vi "room.vi"(7 "conti R3?":bool, 8 "error in (no error)":errorcluster, 9 "Position":T4, 10 "Enum":enum16{"recycle", "box put"}(ring), 11 "main.ctl":T1) -> (0 "error out":errorcluster, 1 "Position out":T4, 3 "main.ctl 2":T1)   [LabVIEW 2019]
uses:
  main data.ctl
  vision/vision_board_ctl.ctl
  block box.ctl
  subVI/move/position cluster.ctl
  servo state.ctl
  route_name.ctl
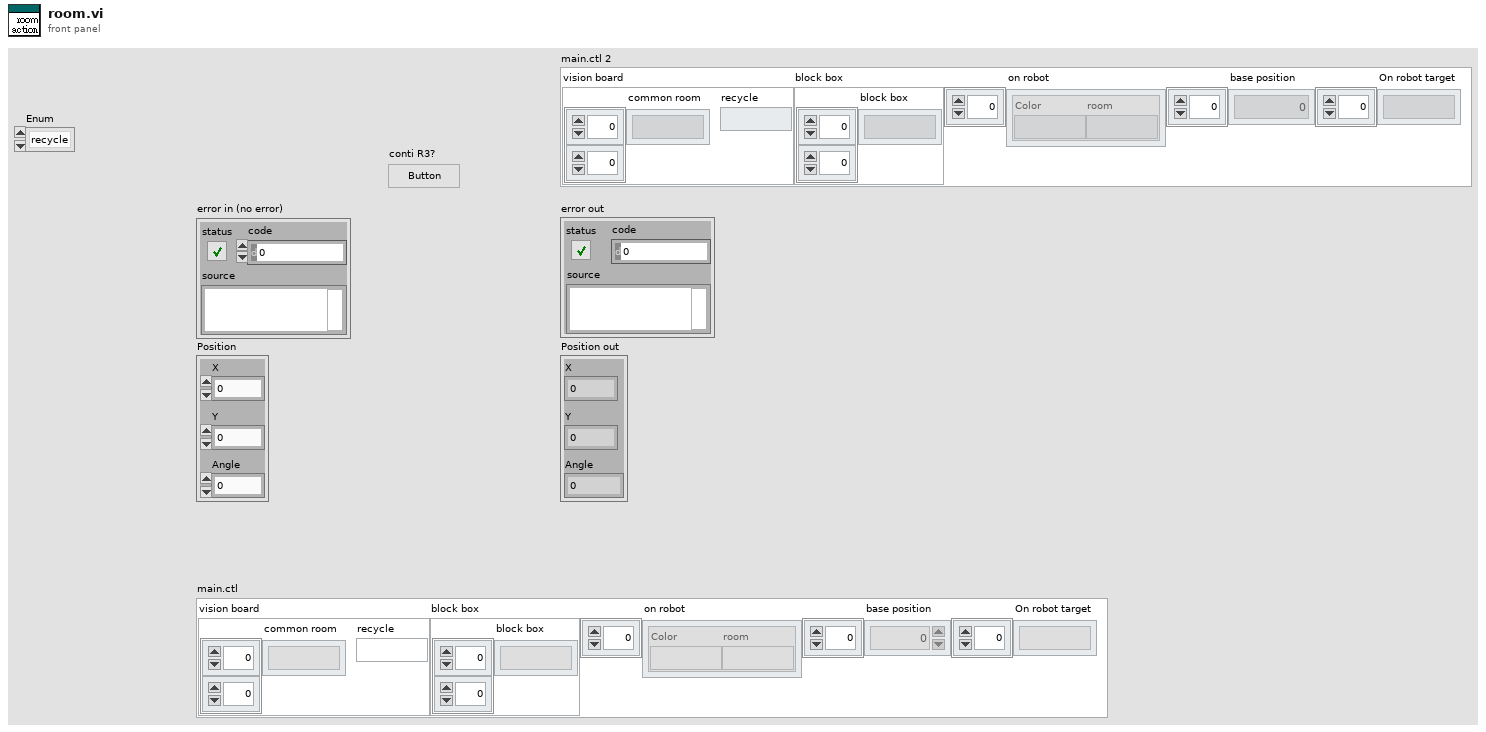
[diagram p1: front panel]
types:
  T1 = typedef "main data.ctl" = cluster{"vision board":T2, "block box":T3, "on robot ":cluster{"Color":string, "room":string}[], "base position":dbl[], "On robot target":string[]}
  T2 = typedef "vision_board_ctl.ctl" = cluster{"common room":string[][], "recycle":string}
  T3 = typedef "block box.ctl" = cluster{"block box":string[][]}
  T4 = typedef "position cluster.ctl" = cluster{"X":dbl, "Y":dbl, "Angle":dbl}
  T5 = typedef "route_name.ctl" = enum16{"S-Vision", "Vision-R1", "Vision-R2", "Vision-R3", "Vision-R4", "Vision-R5", "R1-Vision", "R2-Vision", "R3-Vision", "R4-Vision", "R5-Vision", "Vision-box", "box-recycle", "recycle-box", "box-Vision", "Vision-S", "R2-R3"}
  T6 = typedef "servo state.ctl" = enum16{"catch", "cam-1", "put", "side", "center", "side-2", "put-2"}
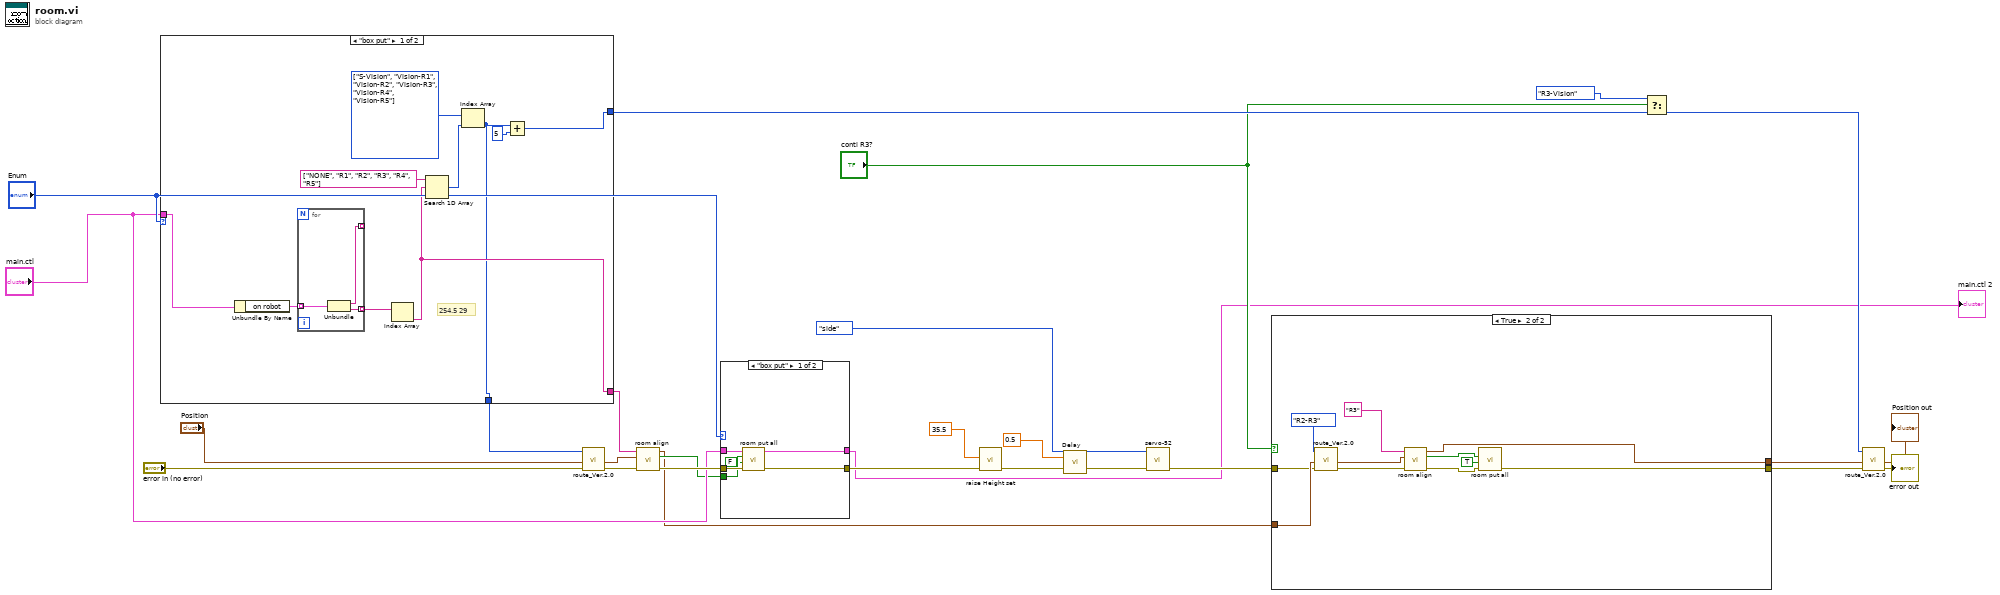
[diagram p0: block diagram]
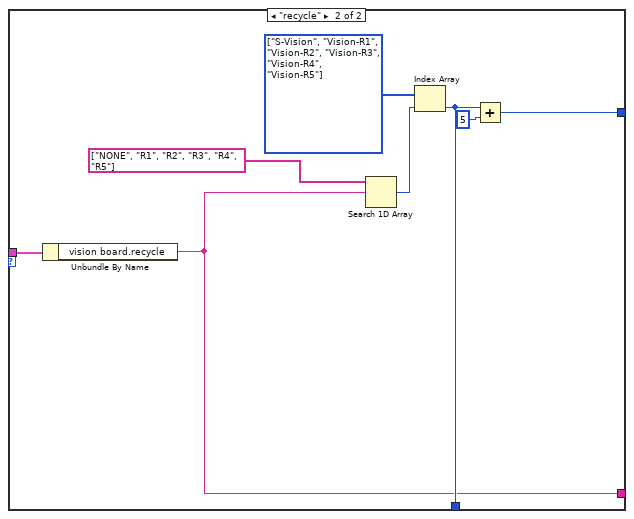
[diagram p3: hidden frame]
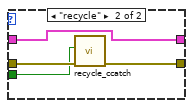
[diagram p4: hidden frame]
diagram:
  n1 = case shown="\"box put\"" "Enum" {
    tunnel: "main.ctl" -> [w28 w45]
    tunnel: [w29 w43] -> w27
    tunnel: [w30 w42] -> w24
    tunnel: [w31 w41] -> w21
    frame "box put" {
      w34 = T5[] [enum."S-Vision", enum."Vision-R1", enum."Vision-R2", enum."Vision-R3", enum."Vision-R4", enum."Vision-R5"] items=["S-Vision", "Vision-R1", "Vision-R2", "Vision-R3", "Vision-R4", "Vision-R5", "R1-Vision", "R2-Vision", "R3-Vision", "R4-Vision", "R5-Vision", "Vision-box", "box-recycle", "recycle-box", "box-Vision", "Vision-S", "R2-R3"]
      # "254.5 29"
      n2 = Unbundle By Name(w28) -> ("on robot"=w37:cluster{"Color":string, "room":string}[])
      n3 = for {
        tunnel: w37 -> [w40] mode=indexing
        tunnel: [w39] -> _ mode=indexing
        tunnel: [w38] -> w36 mode=indexing
        n4 = Unbundle(w40) -> ("Color"=w39:string, "room"=w38:string)
      }
      n5 = Index Array(array=w36) -> (element=w30:string)  [unwired: 1 in]
      n6 = Search 1D Array(1D array=string[] ["NONE", "R1", "R2", "R3", "R4", "R5"], element=w30) -> (index of element=w33:i32)  [unwired: 1 in]
      n7 = Index Array(array=w34, index=w33) -> (element=w29:T5)
      n8 = Add(x=w29, y=5) -> (x+y=w31:i32)
    }
    frame "recycle" {
      w47 = T5[] [enum."S-Vision", enum."Vision-R1", enum."Vision-R2", enum."Vision-R3", enum."Vision-R4", enum."Vision-R5"] items=["S-Vision", "Vision-R1", "Vision-R2", "Vision-R3", "Vision-R4", "Vision-R5", "R1-Vision", "R2-Vision", "R3-Vision", "R4-Vision", "R5-Vision", "Vision-box", "box-recycle", "recycle-box", "box-Vision", "Vision-S", "R2-R3"]
      n9 = Unbundle By Name(w45) -> ("vision board.recycle"=w42:string)
      n10 = Search 1D Array(1D array=string[] ["NONE", "R1", "R2", "R3", "R4", "R5"], element=w42) -> (index of element=w44:i32)  [unwired: 1 in]
      n11 = Index Array(array=w47, index=w44) -> (element=w43:T5)
      n12 = Add(x=w43, y=5) -> (x+y=w41:i32)
    }
  }
  n13 = call "route_Ver.2.0.vi"("error in (no error)"="error in (no error)", "Position"="Position", 11:w27) -> ("error out"=w23:errorcluster, "Position out"=w22:T4)  [unwired: 7 in]
  n14 = call "room align.vi"("error in (no error)"=w23, "Position in"=w22, "recycle"=w24) -> ("error out"=w18:errorcluster, "side?"=w10:bool, "Position out"=w4:T4)  [unwired: 6 in]
  n15 = case shown="\"box put\"" "Enum" {
    tunnel: w18 -> [w54 w58]
    tunnel: [w53 w57] -> w13
    tunnel: "main.ctl" -> [w52 w56]
    tunnel: [w51 w56] -> w1
    tunnel: w10 -> [w50 w55]
    frame "box put" {
      n16 = call "room put all.vi"("error in (no error)"=w54, "R3?"=FALSE, "side?"=w50, "main.ctl"=w52) -> ("error out"=w53:errorcluster, "main.ctl 2"=w51:T1)  [unwired: 6 in]
    }
    frame "recycle" {
      n17 = call "recycle_ccatch.vi"("error in (no error)"=w58, "s"=w55) -> ("error out"=w57:errorcluster)  [unwired: 9 in]
    }
  }
  "main.ctl 2" <- w1
  n18 = call "raise Height set.vi"("error in (no error)"=w13, "Height_cm"=35.5) -> ("error out"=w14:errorcluster)  [unwired: 9 in]
  n19 = call "Delay.vi"("error in (no error)"=w14, "Delay Time (s)"=0.5) -> ("error out"=w11:errorcluster)  [unwired: 1 in]
  n20 = call "servo-52.vi"("error in (no error)"=w11, "Enum"=servo_state."side") -> ("error out"=w8:errorcluster)  [unwired: 9 in]
  n21 = case shown="True" "conti R3?" {
    tunnel: w8 -> [w60 w69]
    tunnel: w4 -> [w59 w70]
    tunnel: [w60 w61] -> w3
    tunnel: [w59 w62] -> w2
    frame False {
    }
    frame True {
      n22 = call "route_Ver.2.0.vi"("error in (no error)"=w69, "Position"=w70, 11:route_name."R2-R3") -> ("error out"=w66:errorcluster, "Position out"=w67:T4)  [unwired: 7 in]
      n23 = call "room align.vi"("error in (no error)"=w66, "Position in"=w67, "recycle"="R3") -> ("error out"=w64:errorcluster, "side?"=w63:bool, "Position out"=w62:T4)  [unwired: 6 in]
      n24 = call "room put all.vi"("error in (no error)"=w64, "R3?"=TRUE, "side?"=w63) -> ("error out"=w61:errorcluster)  [unwired: 7 in, 1 out]
    }
  }
  n25 = Select(t=route_name."R3-Vision", s="conti R3?", f=w21) -> (s? t:f=w7:i32)
  n26 = call "route_Ver.2.0.vi"("error in (no error)"=w3, "Position"=w2, 11:w7) -> ("error out"=→"error out":errorcluster, "Position out"=→"Position out":T4)  [unwired: 7 in]
